vi "Delete Polymorphic.vi"   [LabVIEW 2016, in "Tree Manager.lvclass"]
doc: "Polymorphic instance of the Delete method. Select the appropraite instance to work with or allow this method to adapt automatically."
uses:
  Tree Manager.lvclass
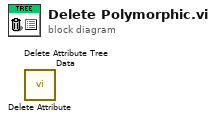
[diagram p0: block diagram]
diagram:
  n1 = call "Delete Attribute.vi"() -> ()  [unwired: 8 in, 4 out]
  n2 = call "Delete Attribute Tree Data.vi"() -> ()  [unwired: 8 in, 4 out]
